vi "带单位测量值字符串.vi"(6 "精度(2)":i16=2, 11 "测量值":dbl) -> (3 "结果":string)   [LabVIEW 2017]
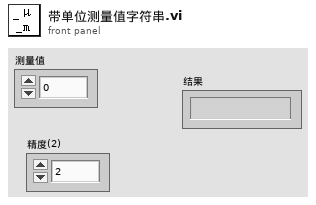
[diagram p1: front panel]
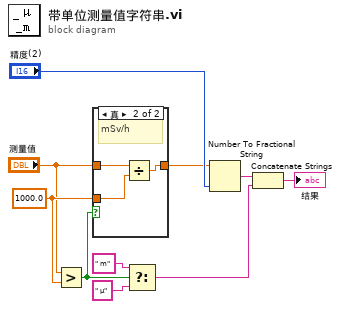
[diagram p0: block diagram]
diagram:
  w8 = 1000.0 ("y")
  n1 = Greater?(x="测量值", y=w8) -> (0:w9:bool)
  n2 = case shown="真" w9 {
    tunnel: "测量值" -> [w11 w14]
    tunnel: w8 -> [_ w13]
    tunnel: [w11 w12] -> w1
    frame False {
      # "uSv/h"
    }
    frame True {
      # "mSv/h"
      n3 = Divide(x=w14, y=w13) -> (x/y=w12:dbl)
    }
  }
  n4 = Select(t=" m" ("F-格式字符串"), s=w9, f=" μ" ("F-格式字符串")) -> (s? t:f=w4:string)
  n5 = Number To Fractional String(number=w1, precision (6)="精度(2)") -> (F-format string=w7:string)  [unwired: 2 in]
  n6 = Concatenate Strings(w7, w4) -> (→"结果":string)
